vi "S2C_VAR_PromptForName.vi"(8 "Error In":errorcluster, 11 "Array?":bool) -> (0 "Error Out":errorcluster, 2 "Size":i32, 3 "Name":string)   [LabVIEW 2015]
panel:
  in  "ArraySize":i32=10 caption="Array Size" min=1 max=250 step=1
  out "Init":bool
  in  "Done":bool
  in  "Text":string caption="Variable Name"
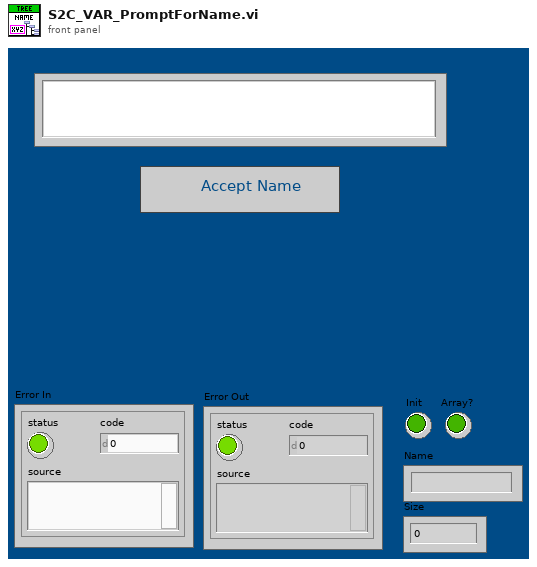
[diagram p1: front panel]
types:
  T1 = cluster{"Selection Start":u32, "Selection End":u32}
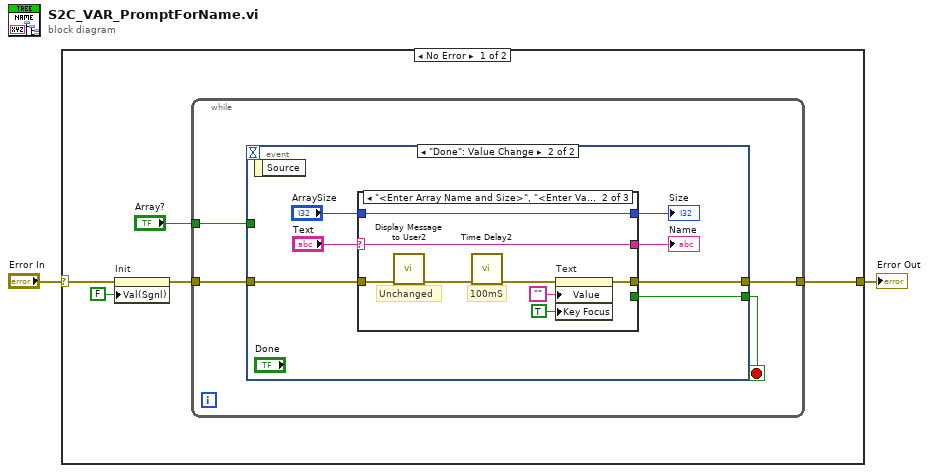
[diagram p0: block diagram]
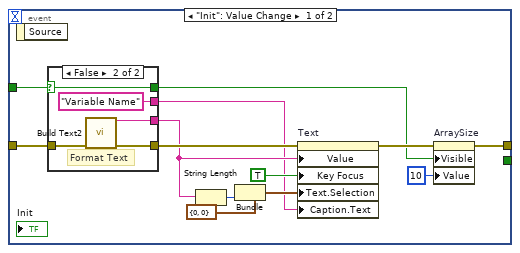
[diagram p2: hidden frame]
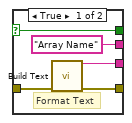
[diagram p3: hidden frame]
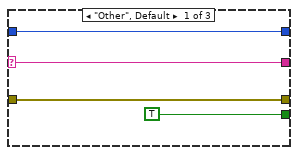
[diagram p4: hidden frame]
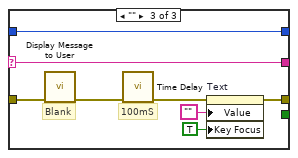
[diagram p5: hidden frame]
diagram:
  n1 = case shown="No Error" "Error In" {
    selector: "Error In" -> [w6 w62]
    tunnel: [w7 w62] -> w1
    frame No Error {
      n2 = property on="Init" class="Bool (strict)"(error in=w6, "Val(Sgnl)"=FALSE ("Value (Signaling)")) -> (error out=w5:errorcluster)  [unwired: 1 in, 1 out]
      n3 = while {
        tunnel: w5 -> [w11]
        tunnel: [w10] -> w7
        tunnel: "Array?" -> [w8]
        stop <- w9 stop-if-true
        n4 = event shown="[1] \"Done\": Value Change" {
          selector: _ -> [_ _]
          dyn-events: _ -> [_ _]
          timeout: _ -> [_ _]
          tunnel: w11 -> [w24 w41]
          tunnel: [w19 w40] -> w10
          tunnel: [_ w37] -> w9
          tunnel: w8 -> [w21 _]
          event "Init": Value Change {
            n5 = event-data() -> ()  [unwired: 1 in, 1 out]
            n6 = case shown="False" w21 {
              selector: w21 -> [w26 w31]
              tunnel: w24 -> [w29 w34]
              tunnel: [w28 w33] -> w23
              tunnel: [w27 w32] -> w15
              tunnel: [w26 w31] -> w17
              tunnel: ["Array Name" "Variable Name"] -> w12
              frame True {
                # "Format Text"
                n7 = call "Build Text"("error in (no error)"=w29) -> ("Result"=w27:string, "error out"=w28:errorcluster)  [unwired: 13 in]
              }
              frame False {
                # "Format Text"
                n8 = call "Build Text2"("error in (no error)"=w34) -> ("Result"=w32:string, "error out"=w33:errorcluster)  [unwired: 13 in]
              }
            }
            n9 = String Length(string=w15) -> (length=w14:i32)
            n10 = Bundle(cluster=T1 {"Selection Start"=0, "Selection End"=0} ("Text.Selection"), "Selection End"=w14) -> (w13:T1)  [unwired: 1 in]
            n11 = property on="Text" class="Str"(error in=w23, "Value"=w15, "Key Focus"=TRUE, "Text.Selection"=w13, "Caption.Text"=w12) -> (error out=w20:errorcluster)  [unwired: 1 in, 1 out]
            n12 = property on="ArraySize" class="DigNum (strict)"(error in=w20, "Visible"=w17, "Value"=10 ("Size")) -> (error out=w19:errorcluster)  [unwired: 1 in, 1 out]
          }
          event "Done": Value Change {
            n13 = event-data() -> ()  [unwired: 1 in, 1 out]
            n14 = case shown="\"<Enter Array Name and Size>\", \"<Enter Variable Name Here>\"" "Text" {
              selector: "Text" -> [w43 w52 w60]
              tunnel: w41 -> [w45 w53 w61]
              tunnel: [w45 w49 w57] -> w40
              tunnel: [w43 w52 w60] -> w38
              tunnel: [TRUE _ _] -> w37
              tunnel: "ArraySize" -> [w42 w46 w54]
              tunnel: [w42 w46 w54] -> w35
              frame "Other", Default {
              }
              frame "<Enter Array Name and Size>", "<Enter Variable Name Here>" {
                # "100mS"
                # "Unchanged"
                n15 = call "Display Message to User2"("error in (no error)"=w53) -> ("error out"=w51:errorcluster)  [unwired: 9 in, 1 out]
                n16 = call "Time Delay2"("error in (no error)"=w51) -> ("error out"=w50:errorcluster)  [unwired: 10 in]
                n17 = property on="Text" class="Str"(error in=w50, "Value"="", "Key Focus"=TRUE) -> (error out=w49:errorcluster)  [unwired: 1 in, 1 out]
              }
              frame "" {
                # "100mS"
                # "Blank"
                n18 = call "Display Message to User"("error in (no error)"=w61) -> ("error out"=w59:errorcluster)  [unwired: 9 in, 1 out]
                n19 = call "Time Delay"("error in (no error)"=w59) -> ("error out"=w58:errorcluster)  [unwired: 10 in]
                n20 = property on="Text" class="Str"(error in=w58, "Value"="", "Key Focus"=TRUE) -> (error out=w57:errorcluster)  [unwired: 1 in, 1 out]
              }
            }
            "Name" <- w38
            "Size" <- w35
          }
        }
      }
    }
    frame Error {
    }
  }
  "Error Out" <- w1
